vi "^Control.vi"   [LabVIEW 2020]
doc: "Control Node\n\nCondition for a Controlled Operation. \nThe target gate is applied ONLY if this control qubit is in the |1> state.\n\nBlock Matrix Structure: [[ 1, 0], [ 0, U]] Where U is the target operation."
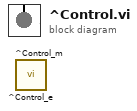
[diagram p0: block diagram]
diagram:
  n1 = call "^Control_e.vi"() -> ()  [unwired: 14 in, 2 out]
  n2 = call "^Control_m.vi"() -> ()  [unwired: 14 in, 2 out]
